vi "Close.vi"(8 "error in (no error)":errorcluster) -> (0 "error out":errorcluster)   [LabVIEW 2015]
uses:
  Display.ctl
  Oscillator.ctl
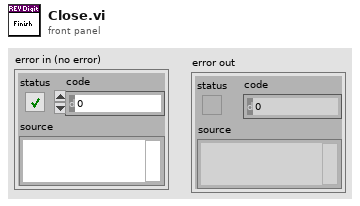
[diagram p1: front panel]
types:
  T1 = typedef "Oscillator.ctl" = enum16{"Off", "On"}
  T2 = typedef "Display.ctl" = enum16{"Off", "On"}
  T3 = typedef "WPI_I2CDevRef.ctl" = cluster{"DevStatus":errorcluster, "Device Address":u8, "Handle":i32, "I2C Bus":T4}
  T4 = typedef "i2c_bus.ctl" = enum16{"I2C On-Board", "I2C MXP", "Invalid"}
  T5 = typedef "WPI_DigitalInputDevRef.ctl" = cluster{"DevStatus":errorcluster, "DIO Channel":T6}
  T6 = typedef "FPGA_DIOChannel.ctl" = enum8{"DIO 0", "DIO 1", "DIO 2", "DIO 3", "DIO 4", "DIO 5", "DIO 6", "DIO 7", "DIO 8", "DIO 9", "DIO MXP 0", "DIO MXP 1", "DIO MXP 2", "DIO MXP 3", "DIO MXP 4", "DIO MXP 5", "DIO MXP 6", "DIO MXP 7", "DIO MXP 8", "DIO MXP 9", "DIO MXP 10", "DIO MXP 11", "DIO MXP 12", "DIO MXP 13", "DIO MXP 14", "DIO MXP 15", "Invalid"}
  T7 = typedef "WPI_AnalogChannelDevRef.ctl" = cluster{"DevStatus":errorcluster, "Analog Channel":T8}
  T8 = typedef "FPGA_AIChannel.ctl" = enum8{"AI 0", "AI 1", "AI 2", "AI 3", "AI MXP 0", "AI MXP 1", "AI MXP 2", "AI MXP 3", "Invalid"}
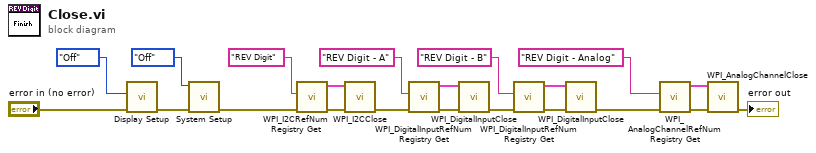
[diagram p0: block diagram]
diagram:
  n1 = call "Display Setup.vi"("error in (no error)"="error in (no error)", "Diplay"=Display."Off") -> ("error out"=w18:errorcluster)  [unwired: 9 in]
  n2 = call "System Setup.vi"("error in (no error)"=w18, "Set Oscillator"=Oscillator."Off") -> ("error out"=w16:errorcluster)  [unwired: 9 in]
  n3 = call <vilib>:"WPI_I2CRefNum Registry Get.vi"("error in (no error)"=w16, "refnum name"="REV Digit") -> ("error out"=w15:errorcluster, "I2CDevRef"=w14:T3)  [unwired: 8 in]
  n4 = call <vilib>:"WPI_I2CClose.vi"("error in (no error)"=w15, "I2CDevRef"=w14) -> ("error out"=w7:errorcluster)  [unwired: 9 in]
  n5 = call <vilib>:"WPI_DigitalInputRefNum Registry Get.vi"("error in (no error)"=w7, "refnum name"="REV Digit - A") -> ("error out"=w9:errorcluster, "DigitalInputDevRef"=w8:T5)  [unwired: 8 in]
  n6 = call <vilib>:"WPI_DigitalInputClose.vi"("error in (no error)"=w9, "DigitalInputDevRef"=w8) -> ("error out"=w5:errorcluster)  [unwired: 9 in]
  n7 = call <vilib>:"WPI_DigitalInputRefNum Registry Get.vi"("error in (no error)"=w5, "refnum name"="REV Digit - B") -> ("error out"=w11:errorcluster, "DigitalInputDevRef"=w10:T5)  [unwired: 8 in]
  n8 = call <vilib>:"WPI_DigitalInputClose.vi"("error in (no error)"=w11, "DigitalInputDevRef"=w10) -> ("error out"=w3:errorcluster)  [unwired: 9 in]
  n9 = call <vilib>:"WPI_AnalogChannelRefNum Registry Get.vi"("error in (no error)"=w3, "refnum name"="REV Digit - Analog") -> ("error out"=w13:errorcluster, "AIDeviceRef"=w12:T7)  [unwired: 8 in]
  n10 = call <vilib>:"WPI_AnalogChannelClose.vi"("error in (no error)"=w13, "AIDeviceRef"=w12) -> ("error out"=→"error out":errorcluster)  [unwired: 9 in]
